vi "Set Report Font.vi"(0 "report in":refnum<class "ooWriter.lvclass">, 1 "text color (unchanged)":u32(colorbox)=16777216, 2 "font settings source":u16(ring) items=["VI Inputs", "Font Dialog Box"], 5 "text options":T2, 9 "font settings":T3={"Charset (-1)"=-1, "Weight (-1)"=-1, "Name"="", "Size"=" "}, 11 "error in (no error)":errorcluster) -> (4 "report out":refnum<class "ooWriter.lvclass">, 6 "font out":T1={"font name"="", "font size"=0.0, "bold"=0, "italic"=0, "underline"=0, "strike through"=0, "font color"=16777216} {"font size" format="%0.2f"; "strike through" items=["Unchanged", "Yes", "No"]; "underline" items=["Unchanged", "Yes", "No"]; "italic" items=["Unchanged", "Yes", "No"]; "bold" items=["Unchanged", "Yes", "No"]}, 15 "error out":errorcluster)   [LabVIEW 2009, in "ooWriter.lvclass"]
doc: "Sets the font properties of the report, including those in the headers and footers."
uses:
  ooWriter.lvclass
  <vilib>/Utility/NIReport.llb/font.ctl
  ooWriter.lvclass/ooWriter.ctl
  C:/Projets/LAVAG/OpenOfficeRGT/AODL/DLLs/AODL.dll
  <vilib>/Utility/NIReport.llb/NI_ReportGenerationCore.lvlib
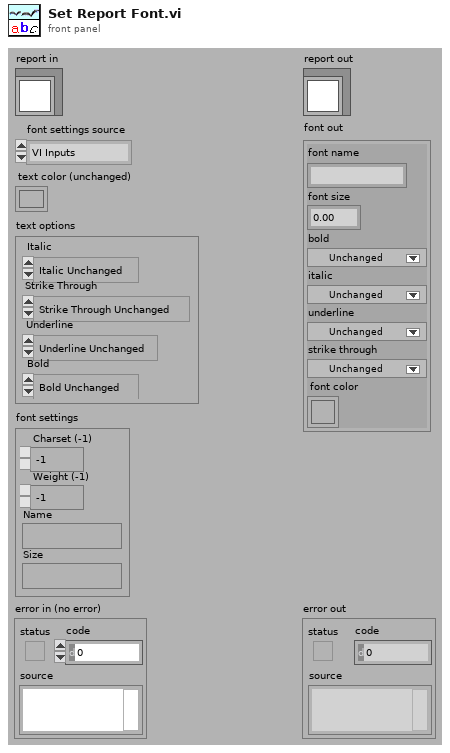
[diagram p1: front panel]
types:
  T1 = typedef "NI_ReportGenerationCore.lvlib/font.ctl" = cluster{"font name":string, "font size":dbl, "bold":u16, "italic":u16, "underline":u16, "strike through":u16, "font color":u32}
  T2 = cluster{"Italic":enum16{"Italic Unchanged", "Italic On", "Italic Off"}, "Strike Through":enum16{"Strike Through Unchanged", "Strike Through On", "Strike Through Off"}, "Underline":enum16{"Underline Unchanged", "Underline On", "Underline Off"}, "Bold":enum16{"Bold Unchanged", "Bold On", "Bold Off"}}
  T3 = cluster{"Charset (-1)":i16, "Weight (-1)":i16, "Name":string, "Size":string}
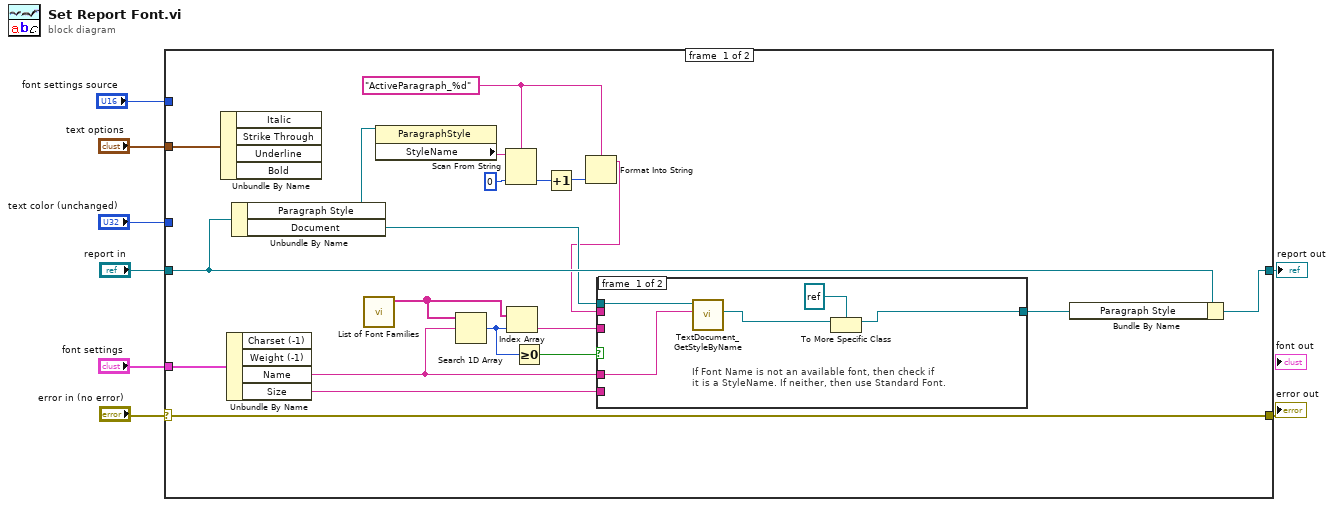
[diagram p0: block diagram]
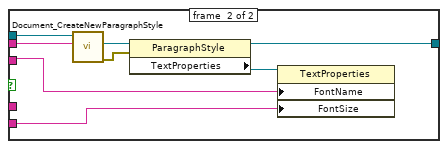
[diagram p2: hidden frame]
diagram:
  n1 = case shown="No Error" "error in (no error)" {
    selector: "error in (no error)" -> [w28 w42]
    tunnel: [w28 w42] -> w8
    tunnel: "report in" -> [w19 w43]
    tunnel: [w18 w43] -> w6
    tunnel: "font settings" -> [w26 _]
    tunnel: "text options" -> [w27 _]
    tunnel: "text color (unchanged)" -> [_ _]
    tunnel: "font settings source" -> [_ _]
    frame #0 {
      w20 = "ActiveParagraph_%d" ("styleName")
      n2 = Unbundle By Name(w27) -> ()  [unwired: 4 out]
      n3 = Unbundle By Name(w26) -> ("Name"=w9:string, "Size"=w10:string)  [unwired: 2 out]
      n4 = Unbundle By Name(w19) -> ("Paragraph Style"=w25:refnum<k24>, "Document"=w14:refnum<k24>)
      n5 = call "List of Font Families.vi"() -> ("Available Fonts"=w17:string[])  [unwired: 11 in]
      n6 = property class="ParagraphStyle"(reference=w25) -> ("StyleName"=w24:string)  [unwired: 1 in, 2 out]
      n7 = Search 1D Array(1D array=w17, element=w9) -> (index of element=w16:i32)  [unwired: 1 in]
      n8 = Scan From String(format string=w20, input string=w24, default 1=0 ("default value 1")) -> (output 1=w22:i32)  [unwired: 2 in, 3 out]
      n9 = Index Array(array=w17, index=w16) -> (element=w11:string)
      n10 = Greater Or Equal To 0?(x=w16) -> (x >= 0?=w15:bool)
      n11 = Increment(x=w22) -> (x+1=w21:i32)
      n12 = Format Into String(format string=w20, w21) -> (resulting string=w12:string)  [unwired: 2 in, 1 out]
      n13 = case shown="False" w15 {
        tunnel: w14 -> [w33 w41]
        tunnel: [w30 w34] -> w13
        tunnel: w12 -> [_ w40]
        tunnel: w11 -> [_ w36]
        tunnel: w10 -> [_ w35]
        tunnel: w9 -> [w29 _]
        frame #0 {
          # "If Font Name is not an available font, then check if\nit is a StyleName. If neither, then use Standard Font."
          n14 = call "TextDocument_GetStyleByName.vi"("StyleName"=w29, "TextDocument in"=w33) -> ("Style"=w32:refnum<k24>)  [unwired: 7 in, 2 out]
          n15 = To More Specific Class(target class=refnum<k24> refnum, reference=w32) -> (specific class reference=w30:refnum<k24>)  [unwired: 1 in, 1 out]
        }
        frame #1 {
          n16 = call "Document_CreateNewParagraphStyle.vi"("styleName"=w40, "document"=w41) -> ("error out"=w38:errorcluster, "Paragraph Style"=w39:refnum<k24>)  [unwired: 7 in, 1 out]
          n17 = property class="ParagraphStyle"(reference=w39, error in=w38) -> (reference out=w34:refnum<k24>, "TextProperties"=w37:refnum<k24>)  [unwired: 1 out]
          n18 = property class="TextProperties"(reference=w37, "FontName"=w36, "FontSize"=w35) -> ()  [unwired: 1 in, 2 out]
        }
      }
      n19 = Bundle By Name(cluster=w19, "Paragraph Style"=w13) -> (w18:refnum<class "ooWriter.lvclass">)
    }
    frame #1 {
    }
  }
  "error out" <- w8
  "report out" <- w6
